vi "Actor Core.vi"(8 "error in":errorcluster, 11 "Nested in":refnum<class "Interactor.lvclass">) -> (0 "error out":errorcluster, 3 "Actor out":refnum<class "Actor.lvclass">)   [LabVIEW 2020, in "Interactor.lvlib" / "Interactor.lvclass"]
doc: "(<B>Filename</B>: Actor Framework.lvlib:Actor.lvclass:Actor Core.vi)\n\nReceives messages to the actor, reacts to them, and initiates any error handling that may shut the actor down.\n\nDescendant classes may override this VI to append parallel tasks for the actor to complete while it handles messages. Overrides use the Call Parent Method node."
uses:
  Interactor.lvclass
  Interactor.lvclass/Interactor.ctl
  Object Dictionary UI/Object Dictionary UI.lvclass
  Home/Home.lvclass
  Network Management UI/Network Management UI.lvclass
  <vilib>/MGI/Panel Manager/Panel/Panel/Subpanel/Subpanel.lvclass
  <vilib>/ActorFramework/Stop Msg/Stop Msg.lvclass
  <vilib>/MGI/Panel Manager/Panel Actor/Panel Actor/Panel Actor.lvclass
  <vilib>/MGI/Panel Manager/Panel/Panel.lvlib
  Interactor Messages/Show Nested Panel Msg/Show Nested Panel Msg.lvclass
  CANopen Master/CANopen Master.lvclass
  Interactor Messages/Publish Discovered Nodes Msg/Publish Discovered Nodes Msg.lvclass
  HAL/Source/Instrument Manager/Instrument Manager.lvclass
  <vilib>/MGI/Panel Manager/Panel/Panel/Subpanel/Subpanel.vi
  <vilib>/MGI/Panel Manager/Panel/Panel Helper/Events.ctl
  <vilib>/MGI/Panel Manager/Panel/Panel Helper/Panel Helper.lvclass
  <vilib>/MGI/Panel Manager/Panel/Panel Helper/Panel Events.ctl
  <vilib>/ActorFramework/Actor/Actor.lvclass
panel:
  in  "NMT":bool
  in  "Copy Log Button":bool
  out "Communication Log":string
  in  "Object Dictionary":bool
  in  "Home Button":bool
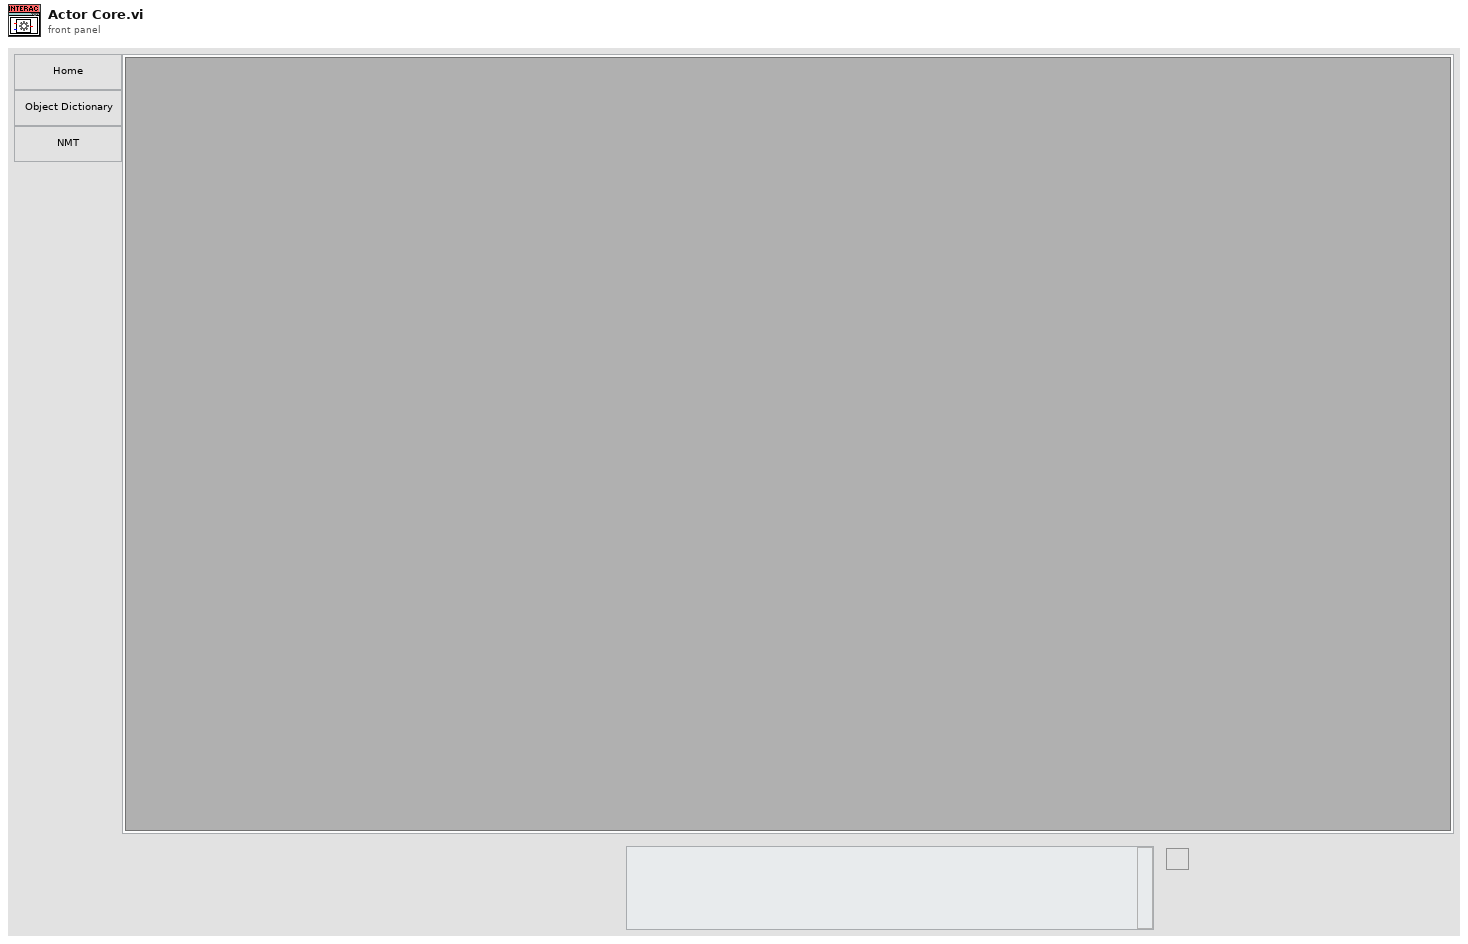
[diagram p1: front panel]
types:
  T1 = cluster{"Pnl Actor":refnum<event-registration>, "Custom":refnum<event-registration>}
  T2 = cluster{"Stop":refnum<user-event>, "Msg Sent Source":refnum<user-event>}
  T3 = cluster{"CAN Task":cluster{"Stop":refnum<user-event>, "Msg Received":refnum<user-event>, "Error":refnum<user-event>}, "NMT":cluster{"Node Discovered":refnum<user-event>}, "Heartbeat Producer":cluster{"Stop":refnum<user-event>, "Error":refnum<user-event>}}
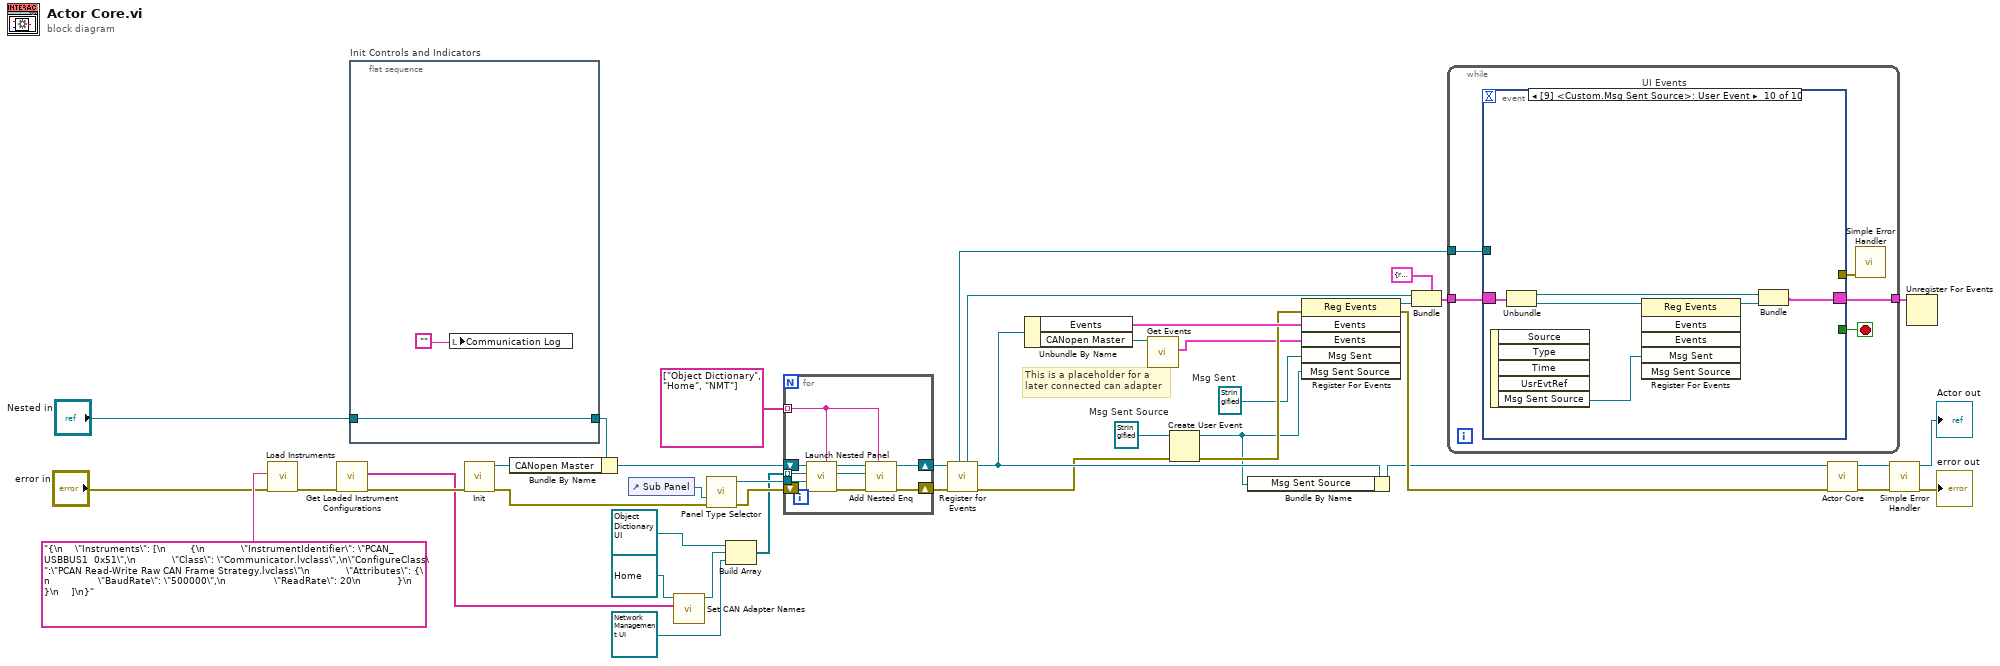
[diagram p0: block diagram]
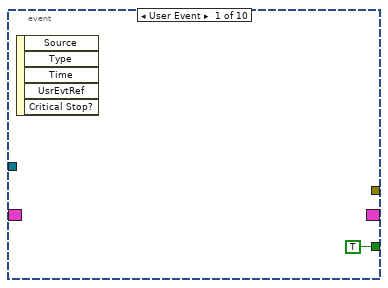
[diagram p2: hidden frame]
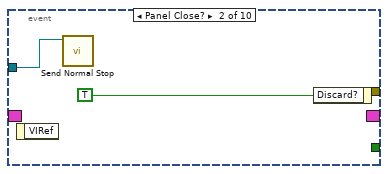
[diagram p3: hidden frame]
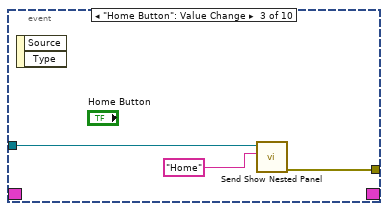
[diagram p4: hidden frame]
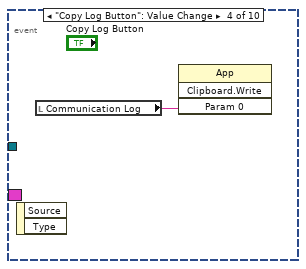
[diagram p5: hidden frame]
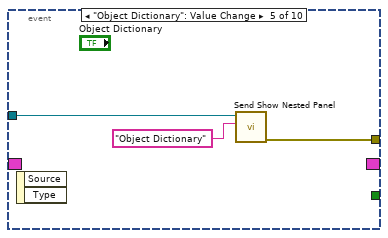
[diagram p6: hidden frame]
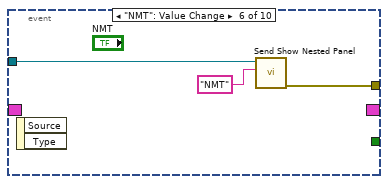
[diagram p7: hidden frame]
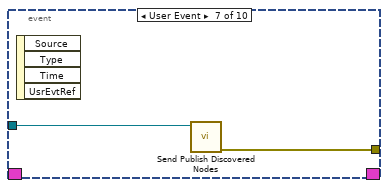
[diagram p8: hidden frame]
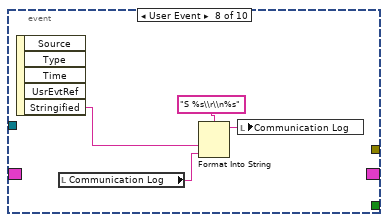
[diagram p9: hidden frame]
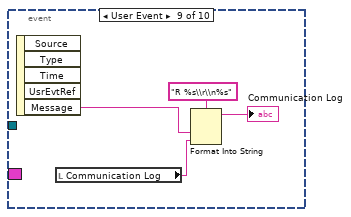
[diagram p10: hidden frame]
diagram:
  w9 = refnum<user-event> refnum  # Msg Sent Source
  w10 = refnum<user-event> refnum  # Msg Sent
  # "This is a placeholder for a\nlater connected can adapter"
  n1 = call "Load Instruments.vi"("Error In"="error in", "Source"="{\n    \"Instruments\": [\n        {\n            \"InstrumentIdentifier\": \"PCAN_USBBUS1  0x51\",\n            \"Class\": \"Communicator.lvclass\",\n\"ConfigureClass\":\"PCAN Read-Write Raw CAN Frame Strategy.lvclass\"\n            \"Attributes\": {\n                \"BaudRate\": \"500000\",\n                \"ReadRate\": 20\n            }\n        }\n    ]\n}" ("<JSON>CFG")) -> ("Error Out"=w13:errorcluster)  [unwired: 9 in]
  n2 = call "Get Loaded Instrument Configurations.vi"("Error In"=w13) -> ("Error Out"=w17:errorcluster, "Identifiers"=w16:string[])  [unwired: 8 in, 1 out]
  n3 = flat-sequence "Init Controls and Indicators" {
    tunnel: "Nested in" -> [w43]
    tunnel: [w43] -> w22
    frame #0 {
      n4 = local write "Communication Log"("") -> ()
    }
  }
  n5 = call "Init.vi"("error in"=w17) -> ("error out"=w19:errorcluster, "CANopen Master out"=w21:refnum<class "CANopen Master.lvclass">)  [unwired: 9 in]
  n6 = Bundle By Name(cluster=w22, "CANopen Master"=w21) -> (w20:refnum<class "Interactor.lvclass">)
  n7 = control-ref of="Sub Panel"() -> (w34:refnum<vi>)
  n8 = call "Set CAN Adapter Names.vi"("ICommunicate Names"=w16, "Home in"=refnum<class "Home.lvclass"> refnum) -> ("Home out"=w26:refnum<class "Home.lvclass">)  [unwired: 9 in]
  n9 = call-poly <vilib>:"Panel Type Selector.vi"("Error In"=w19, "Sub Panel"=w34) -> ("Error Out"=w33:errorcluster, "Subpanel Out"=w29:refnum<class "Subpanel.lvclass">)  [unwired: 8 in]
  n10 = Build Array(refnum<class "Object Dictionary UI.lvclass"> refnum ("Object Dictionary.lvlib:Object Dictionary.lvclass"), w26, refnum<class "Network Management UI.lvclass"> refnum ("Network Management.lvlib:Network Management.lvclass")) -> (w28:refnum<class "Panel Actor.lvclass">[])
  n11 = for {
    tunnel: w29 -> [w46]
    shift-right: [w50] -> w32
    shift-left: w33 -> [w52]
    shift-right: [w47] -> w30
    shift-left: w20 -> [w51]
    tunnel: w28 -> [w45] mode=indexing
    tunnel: string[] ["Object Dictionary", "Home", "NMT"] -> [w44] mode=indexing
    n12 = call <vilib>:"Launch Nested Panel.vi"("Debug Alias"=w44, "error in (no error)"=w52, "Panel"=w46, "Nested Panel Actor"=w45, "Panel Actor in"=w51) -> ("error out"=w50:errorcluster, "Nested Actor's Enqueuer"=w48:refnum<class "Message Enqueuer.lvclass">, "Panel Actor out"=w49:refnum<class "Interactor.lvclass">)  [unwired: 3 in, 1 out]
    n13 = call "Add Nested Enq.vi"("Ident"=w44, "Nested Actor's Enqueuer"=w48, "Interactor in"=w49) -> ("Interactor out"=w47:refnum<class "Interactor.lvclass">)  [unwired: 8 in]
  }
  n14 = call <vilib>:"Register for Events.vi"("Error In"=w32, "Panel Actor in"=w30) -> ("Error Out"=w12:errorcluster, "Panel Actor out"=w31:refnum<class "Interactor.lvclass">, "Pnl Actor"=w35:refnum<event-registration>, "Self Enqueuer"=w38:refnum<class "Message Enqueuer.lvclass">)  [unwired: 6 in]
  n15 = Unbundle By Name(w31) -> ("Events"=w25:T2, "CANopen Master"=w23:refnum<class "CANopen Master.lvclass">)
  n16 = call "Get Events.vi"("CANopen Master in"=w23) -> ("Events"=w2:T3)  [unwired: 9 in, 1 out]
  n17 = Create User Event(user event datatype=w9, error in=w12) -> (user event=w7:refnum<user-event>, error out=w11:errorcluster)
  n18 = Bundle By Name(cluster=w31, "Msg Sent Source"=w7) -> (w8:refnum<class "Interactor.lvclass">)
  n19 = register-events ("Main Register for Events")(error in=w11, w25, w2, w10, w7) -> (reference out=w36:refnum<event-registration>, error out=w24:errorcluster)  [unwired: 1 in]
  n20 = Bundle(cluster=T1 {"Pnl Actor"=refnum, "Custom"=refnum}, "Pnl Actor"=w35, "Custom"=w36) -> (w37:T1)
  n21 = while {
    tunnel: w37 -> [w57]
    tunnel: [w55] -> w39
    tunnel: w38 -> [w54]
    stop <- w56 stop-if-true
    n22 = event "UI Events" shown="[9] <Custom.Msg Sent Source>: User Event" {
      selector: w57 -> [_ _ _ _ _ _ _ _ _ w86]
      dyn-events: [_ _ _ _ _ _ _ _ _ w81] -> w55
      timeout: _ -> [_ _ _ _ _ _ _ _ _ _]
      tunnel: [TRUE _ _ _ _ _ _ _ _ _] -> w56
      tunnel: w54 -> [_ w59 w63 _ w66 w69 w72 _ _ _]
      tunnel: [_ _ w61 _ w65 w68 w71 _ _ _] -> w53
      event User Event {
        n23 = event-data() -> ()  [unwired: 1 in, 5 out]
      }
      event Panel Close? {
        n24 = event-data() -> ()  [unwired: 1 in, 1 out]
        n25 = call <vilib>:"Send Normal Stop.vi"("Message Enqueuer"=w59) -> ()  [unwired: 10 in, 1 out]
        n26 = event-data("Discard?"=TRUE) -> ()  [unwired: 1 in, 1 out]
      }
      event "Home Button": Value Change {
        n27 = event-data() -> ()  [unwired: 1 in, 2 out]
        n28 = call "Send Show Nested Panel.vi"("Ident"="Home", "Message Enqueuer"=w63) -> ("error out"=w61:errorcluster)  [unwired: 8 in, 1 out]
      }
      event "Copy Log Button": Value Change {
        n29 = event-data() -> ()  [unwired: 1 in, 2 out]
        n30 = local read "Communication Log"() -> (w64:string)
        n31 = invoke class="App" method="Clipboard.Write"("Param 0"=w64) -> ()  [unwired: 3 in, 4 out]
      }
      event "Object Dictionary": Value Change {
        n32 = event-data() -> ()  [unwired: 1 in, 2 out]
        n33 = call "Send Show Nested Panel.vi"("Ident"="Object Dictionary", "Message Enqueuer"=w66) -> ("error out"=w65:errorcluster)  [unwired: 8 in, 1 out]
      }
      event "NMT": Value Change {
        n34 = event-data() -> ()  [unwired: 1 in, 2 out]
        n35 = call "Send Show Nested Panel.vi"("Ident"="NMT", "Message Enqueuer"=w69) -> ("error out"=w68:errorcluster)  [unwired: 8 in, 1 out]
      }
      event User Event {
        n36 = event-data() -> ()  [unwired: 1 in, 4 out]
        n37 = call "Send Publish Discovered Nodes.vi"("Message Enqueuer"=w72) -> ("error out"=w71:errorcluster)  [unwired: 9 in, 1 out]
      }
      event User Event {
        n38 = event-data() -> ("Stringified"=w75:string)  [unwired: 1 in, 4 out]
        n39 = local read "Communication Log"() -> (w74:string)
        n40 = Format Into String(format string="S %s\\r\\n%s", w75, w74) -> (resulting string=w73:string)  [unwired: 2 in, 1 out]
        n41 = local write "Communication Log"(w73) -> ()
      }
      event User Event {
        n42 = event-data() -> ("Message"=w80:string)  [unwired: 1 in, 4 out]
        n43 = local read "Communication Log"() -> (w79:string)
        n44 = Format Into String(format string="R %s\\r\\n%s", w80, w79) -> (resulting string=→"Communication Log":string)  [unwired: 2 in, 1 out]
      }
      event User Event {
        n45 = event-data() -> ("Msg Sent Source"=w84:refnum<user-event>)  [unwired: 1 in, 4 out]
        n46 = Unbundle(w86) -> ("Pnl Actor"=w82:refnum<event-registration>, "Custom"=w85:refnum<event-registration>)
        n47 = register-events ("Main Register for Events")(reference=w85, w84) -> (reference out=w83:refnum<event-registration>)  [unwired: 4 in, 1 out]
        n48 = Bundle("Pnl Actor"=w82, "Custom"=w83) -> (w81:T1)  [unwired: 1 in]
      }
    }
    n49 = call <vilib>:"Simple Error Handler.vi"("error in (no error)"=w53) -> ()  [unwired: 4 in, 5 out]
  }
  n50 = call-parent "Actor Core.vi"("error in"=w24, "Panel Actor in"=w8) -> ("error out"=w41:errorcluster, "Actor out"=→"Actor out":refnum<class "Actor.lvclass">)  [unwired: 8 in]
  n51 = call <vilib>:"Simple Error Handler.vi"("error in (no error)"=w41) -> ("error out"=→"error out":errorcluster)  [unwired: 4 in, 4 out]
  n52 = Unregister For Events(event registration refnum=w39) -> ()  [unwired: 1 in, 1 out]
